vi "rsscope_core_global.vi"() -> ()   [LabVIEW 2018] (continued)
None\n\nRemote-control command(s):\nSEARch:TRIGger:HBTO:ERRor:PREamble"}, {"Level"=4, "Class Only"=FALSE, "Identifier"="RSSCOPE_ATTR_SEARCH_100BASE_T1_ERROR_CRC", "Descriptive Name"="Search 100BASE-T1 Error CRC", "Data Type"=3, "Command"="SEAR:TRIG:HBTO:ERR:CRC", "Access"=2, "Range Table"="", "Read Callback"="rsscope_FormatSearchNameBoolean_ReadCallback.vi", "Write Callback"="rsscope_FormatSearchNameBoolean_WriteCallback.vi", "Supported Models"="", "Instrument Options"="K57", "Flags"=0, "Help"="Enables / disables trigger on Cyclic Redundancy Check (CRC) error.\n\nAvailable Repeated Capabilities:\nNone\n\nRemote-control command(s):\nSEARch:TRIGger:HBTO:ERRor:CRC"}, {"Level"=4, "Class Only"=FALSE, "Identifier"="RSSCOPE_ATTR_SEARCH_100BASE_T1_ERROR_SFD", "Descriptive Name"="Search 100BASE-T1 Error SFD", "Data Type"=3, "Command"="SEAR:TRIG:HBTO:ERR:SFD", "Access"=2, "Range Table"="", "Read Callback"="rsscope_FormatSearchNameBoolean_ReadCallback.vi", "Write Callback"="rsscope_FormatSearchNameBoolean_WriteCallback.vi", "Supported Models"="", "Instrument Options"="K57", "Flags"=0, "Help"="Enables / disables search for start frame delimiter (SFD) error.\n\nAvailable Repeated Capabilities:\nNone\n\nRemote-control command(s):\nSEARch:TRIGger:HBTO:ERRor:SFD"}, {"Level"=4, "Class Only"=TRUE, "Identifier"="", "Descriptive Name"="Results", "Data Type"=0, "Command"="", "Access"=0, "Range Table"="", "Read Callback"="", "Write Callback"="", "Supported Models"="", "Instrument Options"="", "Flags"=0, "Help"="Returns the search results."}, {"Level"=5, "Class Only"=FALSE, "Identifier"="RSSCOPE_ATTR_SEARCH_100BASE_T1_FRAME_COUNT", "Descriptive Name"="Search 100BASE-T1 Frame Count", "Data Type"=0, "Command"="SEAR:RES:HBTO:FCO?", "Access"=0, "Range Table"="", "Read Callback"="rsscope_FormatSearchNameInt32_ReadCallback.vi", "Write Callback"="", "Supported Models"="", "Instrument Options"="K57", "Flags"=0, "Help"="Returns the number of decoded frames within the search result.\n\nAvailable Repeated Capabilities:\nNone\n\nRemote-control command(s):\nSEARch:RESult:HBTO:FCOunt?"}, {"Level"=3, "Class Only"=TRUE, "Identifier"="", "Descriptive Name"="1000BASE-T1", "Data Type"=0, "Command"="", "Access"=0, "Range Table"="", "Read Callback"="", "Write Callback"="", "Supported Models"="", "Instrument Options"="", "Flags"=0, "Help"="Configures 1000BASE-T1 search"}, {"Level"=4, "Class Only"=FALSE, "Identifier"="RSSCOPE_ATTR_SEARCH_1000BASE_T1_TYPE", "Descriptive Name"="Search 1000BASE-T1 Type", "Data Type"=0, "Command"="SEAR:TRIG:TBTO:TYPE", "Access"=2, "Range Table"="RsScope_rngSearch1000BASE_T1Type", "Read Callback"="rsscope_FormatSearchNameInt32_ReadCallback.vi", "Write Callback"="rsscope_FormatSearchNameInt32_WriteCallback.vi", "Supported Models"="", "Instrument Options"="K58", "Flags"=0, "Help"="Selects the type of frame to be searched for.\n\nAvailable Repeated Capabilities:\nNone\n\nRemote-control command(s):\nSEARch:TRIGger:TBTO:TYPE"}, {"Level"=4, "Class Only"=FALSE, "Identifier"="RSSCOPE_ATTR_SEARCH_1000BASE_T1_DESTINATION_ADDRESS_CONDITION", "Descriptive Name"="Search 1000BASE-T1 Destination Address Condition", "Data Type"=0, "Command"="SEAR:TRIG:TBTO:DADD:COND", "Access"=2, "Range Table"="rsscope_rngProtocolTriggerConditionStrict", "Read Callback"="rsscope_FormatSearchNameInt32_ReadCallback.vi", "Write Callback"="rsscope_FormatSearchNameInt32_WriteCallback.vi", "Supported Models"="", "Instrument Options"="K58", "Flags"=0, "Help"="Sets the condition for the destination address. You can define an exact value or a value range.\n\nAvailable Repeated Capabilities:\nNone\n\nRemote-control command(s):\nSEARch:TRIGger:TBTO:DADDress:CONDition"}, {"Level"=4, "Class Only"=FALSE, "Identifier"="RSSCOPE_ATTR_SEARCH_1000BASE_T1_DESTINATION_ADDRESS_MIN", "Descriptive Name"="Search 1000BASE-T1 Destination Address Min", "Data Type"=2, "Command"="SEAR:TRIG:TBTO:DADD:MIN", "Access"=2, "Range Table"="", "Read Callback"="rsscope_FormatSearchNameString_ReadCallback.vi", "Write Callback"="rsscope_FormatSearchNameString_WriteCallback.vi", "Supported Models"="", "Instrument Options"="K58", "Flags"=0, "Help"="Specifies the destination address bit pattern, or sets the start value of a pattern range. The string parameter accepts the bit value X (do not care).\n\nAvailable Repeated Capabilities:\nNone\n\nRemote-control command(s):\nSEARch:TRIGger:TBTO:DADDress:MIN"}, {"Level"=4, "Class Only"=FALSE, "Identifier"="RSSCOPE_ATTR_SEARCH_1000BASE_T1_DESTINATION_ADDRESS_MAX", "Descriptive Name"="Search 1000BASE-T1 Destination Address Max", "Data Type"=2, "Command"="SEAR:TRIG:TBTO:DADD:MAX", "Access"=2, "Range Table"="", "Read Callback"="rsscope_FormatSearchNameString_ReadCallback.vi", "Write Callback"="rsscope_FormatSearchNameString_WriteCallback.vi", "Supported Models"="", "Instrument Options"="K58", "Flags"=0, "Help"="Sets the end value of the destination address range if RSSCOPE_ATTR_SEARCH_1000BASE_T1_DESTINATION_ADDRESS_CONDITION is set to In Range or Out Of Range. The string parameter accepts the bit value X (do not care).\n\nAvailable Repeated Capabilities:\nNone\n\nRemote-control command(s):\nSEARch:TRIGger:TBTO:DADDress:MAX"}, {"Level"=4, "Class Only"=FALSE, "Identifier"="RSSCOPE_ATTR_SEARCH_1000BASE_T1_SOURCE_ADDRESS_CONDITION", "Descriptive Name"="Search 1000BASE-T1 Source Address Condition", "Data Type"=0, "Command"="SEAR:TRIG:TBTO:SADD:COND", "Access"=2, "Range Table"="rsscope_rngProtocolTriggerConditionStrict", "Read Callback"="rsscope_FormatSearchNameInt32_ReadCallback.vi", "Write Callback"="rsscope_FormatSearchNameInt32_WriteCallback.vi", "Supported Models"="", "Instrument Options"="K58", "Flags"=0, "Help"="Sets the condition for the source address. You can define an exact value or a value range.\n\nAvailable Repeated Capabilities:\nNone\n\nRemote-control command(s):\nSEARch:TRIGger:TBTO:SADDress:CONDition"}, {"Level"=4, "Class Only"=FALSE, "Identifier"="RSSCOPE_ATTR_SEARCH_1000BASE_T1_SOURCE_ADDRESS_MIN", "Descriptive Name"="Search 1000BASE-T1 Source Address Min", "Data Type"=2, "Command"="SEAR:TRIG:TBTO:SADD:MIN", "Access"=2, "Range Table"="", "Read Callback"="rsscope_FormatSearchNameString_ReadCallback.vi", "Write Callback"="rsscope_FormatSearchNameString_WriteCallback.vi", "Supported Models"="", "Instrument Options"="K58", "Flags"=0, "Help"="Specifies the source address bit pattern, or sets the start value of a pattern range. The string parameter accepts the bit value X (do not care).\n\nAvailable Repeated Capabilities:\nNone\n\nRemote-control command(s):\nSEARch:TRIGger:TBTO:SADDress:MIN"}, {"Level"=4, "Class Only"=FALSE, "Identifier"="RSSCOPE_ATTR_SEARCH_1000BASE_T1_SOURCE_ADDRESS_MAX", "Descriptive Name"="Search 1000BASE-T1 Source Address Max", "Data Type"=2, "Command"="SEAR:TRIG:TBTO:SADD:MAX", "Access"=2, "Range Table"="", "Read Callback"="rsscope_FormatSearchNameString_ReadCallback.vi", "Write Callback"="rsscope_FormatSearchNameString_WriteCallback.vi", "Supported Models"="", "Instrument Options"="K58", "Flags"=0, "Help"="Sets the end value of the source address range if RSSCOPE_ATTR_SEARCH_1000BASE_T1_SOURCE_ADDRESS_CONDITION is set to In Range or Out Of Range. The string parameter accepts the bit value X (do not care).\n\nAvailable Repeated Capabilities:\nNone\n\nRemote-control command(s):\nSEARch:TRIGger:TBTO:SADDress:MAX"}, {"Level"=4, "Class Only"=FALSE, "Identifier"="RSSCOPE_ATTR_SEARCH_1000BASE_T1_LENGTH_TYPE_CONDITION", "Descriptive Name"="Search 1000BASE-T1 Length Type Condition", "Data Type"=0, "Command"="SEAR:TRIG:TBTO:LENG:COND", "Access"=2, "Range Table"="rsscope_rngProtocolTriggerConditionStrict", "Read Callback"="rsscope_FormatSearchNameInt32_ReadCallback.vi", "Write Callback"="rsscope_FormatSearchNameInt32_WriteCallback.vi", "Supported Models"="", "Instrument Options"="K58", "Flags"=0, "Help"="Sets the condition for the length/type. You can define an exact value or a value range.\n\nAvailable Repeated Capabilities:\nNone\n\nRemote-control command(s):\nSEARch:TRIGger:TBTO:LENGth:CONDition"}, {"Level"=4, "Class Only"=FALSE, "Identifier"="RSSCOPE_ATTR_SEARCH_1000BASE_T1_LENGTH_TYPE_MIN", "Descriptive Name"="Search 1000BASE-T1 Length Type Min", "Data Type"=2, "Command"="SEAR:TRIG:TBTO:LENG:MIN", "Access"=2, "Range Table"="", "Read Callback"="rsscope_FormatSearchNameString_ReadCallback.vi", "Write Callback"="rsscope_FormatSearchNameString_WriteCallback.vi", "Supported Models"="", "Instrument Options"="K58", "Flags"=0, "Help"="Specifies the length/ type bit pattern, or sets the start value of a pattern range. The string parameter accepts the bit value X (do not care).\n\nAvailable Repeated Capabilities:\nNone\n\nRemote-control command(s):\nSEARch:TRIGger:TBTO:LENGth:MIN"}, {"Level"=4, "Class Only"=FALSE, "Identifier"="RSSCOPE_ATTR_SEARCH_1000BASE_T1_LENGTH_TYPE_MAX", "Descriptive Name"="Search 1000BASE-T1 Length Type Max", "Data Type"=2, "Command"="SEAR:TRIG:TBTO:LENG:MAX", "Access"=2, "Range Table"="", "Read Callback"="rsscope_FormatSearchNameString_ReadCallback.vi", "Write Callback"="rsscope_FormatSearchNameString_WriteCallback.vi", "Supported Models"="", "Instrument Options"="K58", "Flags"=0, "Help"="Sets the end value of the length/type range if RSSCOPE_ATTR_SEARCH_1000BASE_T1_TYPE_LENGTH_CONDITION is set to In Range or Out Of Range. The string parameter accepts the bit value X (do not care).\n\nAvailable Repeated Capabilities:\nNone\n\nRemote-control command(s):\nSEARch:TRIGger:TBTO:LENGth:MAX"}, {"Level"=4, "Class Only"=FALSE, "Identifier"="RSSCOPE_ATTR_SEARCH_1000BASE_T1_FRAME_CHECK_CRC_CONDITION", "Descriptive Name"="Search 1000BASE-T1 Frame Check CRC Condition", "Data Type"=0, "Command"="SEAR:TRIG:TBTO:CRC:COND", "Access"=2, "Range Table"="rsscope_rngProtocolTriggerConditionStrict", "Read Callback"="rsscope_FormatSearchNameInt32_ReadCallback.vi", "Write Callback"="rsscope_FormatSearchNameInt32_WriteCallback.vi", "Supported Models"="", "Instrument Options"="K58", "Flags"=0, "Help"="Sets the condition for the frame check. You can define an exact value or a value range.\n\nAvailable Repeated Capabilities:\nNone\n\nRemote-control command(s):\nSEARch:TRIGger:TBTO:CRC:CONDition"}, {"Level"=4, "Class Only"=FALSE, "Identifier"="RSSCOPE_ATTR_SEARCH_1000BASE_T1_FRAME_CHECK_CRC_MIN", "Descriptive Name"="Search 1000BASE-T1 Frame Check CRC Min", "Data Type"=2, "Command"="SEAR:TRIG:TBTO:CRC:MIN", "Access"=2, "Range Table"="", "Read Callback"="rsscope_FormatSearchNameString_ReadCallback.vi", "Write Callback"="rsscope_FormatSearchNameString_WriteCallback.vi", "Supported Models"="", "Instrument Options"="K58", "Flags"=0, "Help"="Specifies the frame check bit pattern, or sets the start value of a pattern range. The string parameter accepts the bit value X (do not care).\n\nAvailable Repeated Capabilities:\nNone\n\nRemote-control command(s):\nSEARch:TRIGger:TBTO:CRC:MIN"}, {"Level"=4, "Class Only"=FALSE, "Identifier"="RSSCOPE_ATTR_SEARCH_1000BASE_T1_FRAME_CHECK_CRC_MAX", "Descriptive Name"="Search 1000BASE-T1 Frame Check CRC Max", "Data Type"=2, "Command"="SEAR:TRIG:TBTO:CRC:MAX", "Access"=2, "Range Table"="", "Read Callback"="rsscope_FormatSearchNameString_ReadCallback.vi", "Write Callback"="rsscope_FormatSearchNameString_WriteCallback.vi", "Supported Models"="", "Instrument Options"="K58", "Flags"=0, "Help"="Sets the end value of the frame check range if RSSCOPE_ATTR_SEARCH_1000BASE_T1_CRC_CONDITION is set to In Range or Out Of Range. The string parameter accepts the bit value X (do not care).\n\nAvailable Repeated Capabilities:\nNone\n\nRemote-control command(s):\nSEARch:TRIGger:TBTO:CRC:MAX"}, {"Level"=4, "Class Only"=FALSE, "Identifier"="RSSCOPE_ATTR_SEARCH_1000BASE_T1_DATA_CONDITION", "Descriptive Name"="Search 1000BASE-T1 Data Condition", "Data Type"=0, "Command"="SEAR:TRIG:TBTO:DATA:DCON", "Access"=2, "Range Table"="rsscope_rngProtocolTriggerConditionStrict", "Read Callback"="rsscope_FormatSearchNameInt32_ReadCallback.vi", "Write Callback"="rsscope_FormatSearchNameInt32_WriteCallback.vi", "Supported Models"="", "Instrument Options"="K58", "Flags"=0, "Help"="Sets the condition for the data. You can define an exact value or a value range.\n\nAvailable Repeated Capabilities:\nNone\n\nRemote-control command(s):\nSEARch:TRIGger:TBTO:DATA:DCONdition"}, {"Level"=4, "Class Only"=FALSE, "Identifier"="RSSCOPE_ATTR_SEARCH_1000BASE_T1_DATA_MIN", "Descriptive Name"="Search 1000BASE-T1 Data Min", "Data Type"=2, "Command"="SEAR:TRIG:TBTO:DATA:DMIN", "Access"=2, "Range Table"="", "Read Callback"="rsscope_FormatSearchNameString_ReadCallback.vi", "Write Callback"="rsscope_FormatSearchNameString_WriteCallback.vi", "Supported Models"="", "Instrument Options"="K58", "Flags"=0, "Help"="Specifies the data bit pattern, or sets the start value of a pattern range. The string parameter accepts the bit value X (do not care).\n\nAvailable Repeated Capabilities:\nNone\n\nRemote-control command(s):\nSEARch:TRIGger:TBTO:DATA:DMIN"}, {"Level"=4, "Class Only"=FALSE, "Identifier"="RSSCOPE_ATTR_SEARCH_1000BASE_T1_DATA_MAX", "Descriptive Name"="Search 1000BASE-T1 Data Max", "Data Type"=2, "Command"="SEAR:TRIG:TBTO:DATA:DMAX", "Access"=2, "Range Table"="", "Read Callback"="rsscope_FormatSearchNameString_ReadCallback.vi", "Write Callback"="rsscope_FormatSearchNameString_WriteCallback.vi", "Supported Models"="", "Instrument Options"="K58", "Flags"=0, "Help"="Sets the end value of the data range if RSSCOPE_ATTR_SEARCH_1000BASE_T1_DATA_CONDITION is set to In Range or Out Of Range. The string parameter accepts the bit value X (do not care).\n\nAvailable Repeated Capabilities:\nNone\n\nRemote-control command(s):\nSEARch:TRIGger:TBTO:DATA:DMAX"}, {"Level"=4, "Class Only"=FALSE, "Identifier"="RSSCOPE_ATTR_SEARCH_1000BASE_T1_INDEX_CONDITION", "Descriptive Name"="Search 1000BASE-T1 Index Condition", "Data Type"=0, "Command"="SEAR:TRIG:TBTO:DATA:ICON", "Access"=2, "Range Table"="rsscope_rngProtocolTriggerConditionStrict", "Read Callback"="rsscope_FormatSearchNameInt32_ReadCallback.vi", "Write Callback"="rsscope_FormatSearchNameInt32_WriteCallback.vi", "Supported Models"="", "Instrument Options"="K58", "Flags"=0, "Help"="Sets the search condition for the index. You can define an exact value or a value range.\n\nAvailable Repeated Capabilities:\nNone\n\nRemote-control command(s):\nSEARch:TRIGger:TBTO:DATA:ICONdition"}, {"Level"=4, "Class Only"=FALSE, "Identifier"="RSSCOPE_ATTR_SEARCH_1000BASE_T1_INDEX_MIN", "Descriptive Name"="Search 1000BASE-T1 Index Min", "Data Type"=0, "Command"="SEAR:TRIG:TBTO:DATA:IMIN", "Access"=2, "Range Table"="RsScope_rng1000BASET1Index", "Read Callback"="rsscope_FormatSearchNameInt32_ReadCallback.vi", "Write Callback"="rsscope_FormatSearchNameInt32_WriteCallback.vi", "Supported Models"="", "Instrument Options"="K58", "Flags"=0, "Help"="Specifies the index bit pattern, or sets the start value of a pattern range.\n\nAvailable Repeated Capabilities:\nNone\n\nRemote-control command(s):\nSEARch:TRIGger:TBTO:DATA:IMIN"}, {"Level"=4, "Class Only"=FALSE, "Identifier"="RSSCOPE_ATTR_SEARCH_1000BASE_T1_INDEX_MAX", "Descriptive Name"="Search 1000BASE-T1 Index Max", "Data Type"=0, "Command"="SEAR:TRIG:TBTO:DATA:IMAX", "Access"=2, "Range Table"="RsScope_rng1000BASET1Index", "Read Callback"="rsscope_FormatSearchNameInt32_ReadCallback.vi", "Write Callback"="rsscope_FormatSearchNameInt32_WriteCallback.vi", "Supported Models"="", "Instrument Options"="K58", "Flags"=0, "Help"="Sets the end value of the index range to be searched for, if RSSCOPE_ATTR_SEARCH_1000BASE_T1_INDEX_CONDITION is set to In Range or Out Of Range.\n\nAvailable Repeated Capabilities:\nNone\n\nRemote-control command(s):\nSEARch:TRIGger:TBTO:DATA:IMAX"}, {"Level"=4, "Class Only"=FALSE, "Identifier"="RSSCOPE_ATTR_SEARCH_1000BASE_T1_ERROR_RS_FEC", "Descriptive Name"="Search 1000BASE-T1 Error RS-FEC", "Data Type"=3, "Command"="SEAR:TRIG:TBTO:ERR:FEC", "Access"=2, "Range Table"="", "Read Callback"="rsscope_FormatSearchNameBoolean_ReadCallback.vi", "Write Callback"="rsscope_FormatSearchNameBoolean_WriteCallback.vi", "Supported Models"="", "Instrument Options"="K58", "Flags"=0, "Help"="Enables search for RS-FEC errors.\n\nAvailable Repeated Capabilities:\nNone\n\nRemote-control command(s):\nSEARch:TRIGger:TBTO:ERRor:FEC"}, {"Level"=4, "Class Only"=FALSE, "Identifier"="RSSCOPE_ATTR_SEARCH_1000BASE_T1_ERROR_CRC", "Descriptive Name"="Search 1000BASE-T1 Error CRC", "Data Type"=3, "Command"="SEAR:TRIG:TBTO:ERR:CRC", "Access"=2, "Range Table"="", "Read Callback"="rsscope_FormatSearchNameBoolean_ReadCallback.vi", "Write Callback"="rsscope_FormatSearchNameBoolean_WriteCallback.vi", "Supported Models"="", "Instrument Options"="K58", "Flags"=0, "Help"="Enables search for cyclic redundancy check (CRC) error.\n\nAvailable Repeated Capabilities:\nNone\n\nRemote-control command(s):\nSEARch:TRIGger:TBTO:ERRor:CRC"}, {"Level"=4, "Class Only"=FALSE, "Identifier"="RSSCOPE_ATTR_SEARCH_1000BASE_T1_ERROR_OUT_OF_RANGE", "Descriptive Name"="Search 1000BASE-T1 Error Out Of Range", "Data Type"=3, "Command"="SEAR:TRIG:TBTO:ERR:OOR", "Access"=2, "Range Table"="", "Read Callback"="rsscope_FormatSearchNameBoolean_ReadCallback.vi", "Write Callback"="rsscope_FormatSearchNameBoolean_WriteCallback.vi", "Supported Models"="", "Instrument Options"="K58", "Flags"=0, "Help"="Enables search for values that are out of range.\n\nAvailable Repeated Capabilities:\nNone\n\nRemote-control command(s):\nSEARch:TRIGger:TBTO:ERRor:OOR"}, {"Level"=4, "Class Only"=FALSE, "Identifier"="RSSCOPE_ATTR_SEARCH_1000BASE_T1_ERROR_ZERO_TERNARY_SYMBOL", "Descriptive Name"="Search 1000BASE-T1 Error Zero Ternary Symbol", "Data Type"=3, "Command"="SEAR:TRIG:TBTO:ERR:ZERO", "Access"=2, "Range Table"="", "Read Callback"="rsscope_FormatSearchNameBoolean_ReadCallback.vi", "Write Callback"="rsscope_FormatSearchNameBoolean_WriteCallback.vi", "Supported Models"="", "Instrument Options"="K58", "Flags"=0, "Help"="Enables search for zero ternary symbol pairs error.\n\nAvailable Repeated Capabilities:\nNone\n\nRemote-control command(s):\nSEARch:TRIGger:TBTO:ERRor:ZERO"}, {"Level"=4, "Class Only"=TRUE, "Identifier"="", "Descriptive Name"="Results", "Data Type"=0, "Command"="", "Access"=0, "Range Table"="", "Read Callback"="", "Write Callback"="", "Supported Models"="", "Instrument Options"="", "Flags"=0, "Help"="Returns the search results."}, {"Level"=5, "Class Only"=FALSE, "Identifier"="RSSCOPE_ATTR_SEARCH_1000BASE_T1_FRAME_COUNT", "Descriptive Name"="Search 1000BASE-T1 Frame Count", "Data Type"=0, "Command"="SEAR:RES:TBTO:FCO?", "Access"=0, "Range Table"="", "Read Callback"="rsscope_FormatSearchNameInt32_ReadCallback.vi", "Write Callback"="", "Supported Models"="", "Instrument Options"="K58", "Flags"=0, "Help"="Returns the number of decoded frames within the search result.\n\nAvailable Repeated Capabilities:\nNone\n\nRemote-control command(s):\nSEARch:RESult:TBTO:FCOunt?"}, {"Level"=5, "Class Only"=FALSE, "Identifier"="RSSCOPE_ATTR_SEARCH_1000BASE_T1_SELECTED_FRAME", "Descriptive Name"="Search 1000BASE-T1 Selected Frame", "Data Type"=0, "Command"="", "Access"=2, "Range Table"="", "Read Callback"="", "Write Callback"="", "Supported Models"="", "Instrument Options"="K58", "Flags"=0, "Help"="Sets the selector for the Frame repeated capability.\n\nAvailable Repeated Capabilities:\nNone\n\nRemote-control command(s):\n"}, {"Level"=5, "Class Only"=FALSE, "Identifier"="RSSCOPE_ATTR_SEARCH_1000BASE_T1_FRAME_STATUS", "Descriptive Name"="Search 1000BASE-T1 Frame Status", "Data Type"=0, "Command"="SEAR:RES:TBTO:FRAM<Frame>:STAT?", "Access"=0, "Range Table"="RsScope_rngProtocol1000BASE_T1FrameStatus", "Read Callback"="rsscope_FormatSearchNameTBTOFrameInt32_ReadCallback.vi", "Write Callback"="", "Supported Models"="", "Instrument Options"="K58", "Flags"=0, "Help"="Returns the state of the frame within the search result.\n\nAvailable Repeated Capabilities:\nNone\n\nRemote-control command(s):\nSEARch:RESult:TBTO:FRAMe<m>:STATe?"}, {"Level"=5, "Class Only"=FALSE, "Identifier"="RSSCOPE_ATTR_SEARCH_1000BASE_T1_FRAME_START_TIME", "Descriptive Name"="Search 1000BASE-T1 Frame Start Time", "Data Type"=1, "Command"="SEAR:RES:TBTO:FRAM<Frame>:STAR?", "Access"=0, "Range Table"="", "Read Callback"="rsscope_FormatSearchNameTBTOFrameReal64_ReadCallback.vi", "Write Callback"="", "Supported Models"="", "Instrument Options"="K58", "Flags"=0, "Help"="Returns the start time of the selected frame within the search result.\n\nAvailable Repeated Capabilities:\nNone\n\nRemote-control command(s):\nSEARch:RESult:TBTO:FRAMe<m>:STARt?"}, {"Level"=5, "Class Only"=FALSE, "Identifier"="RSSCOPE_ATTR_SEARCH_1000BASE_T1_FRAME_STOP_TIME", "Descriptive Name"="Search 1000BASE-T1 Frame Stop Time", "Data Type"=1, "Command"="SEAR:RES:TBTO:FRAM<Frame>:STOP?", "Access"=0, "Range Table"="", "Read Callback"="rsscope_FormatSearchNameTBTOFrameReal64_ReadCallback.vi", "Write Callback"="", "Supported Models"="", "Instrument Options"="K58", "Flags"=0, "Help"="Returns the end time of the selected frame within the search result.\n\nAvailable Repeated Capabilities:\nNone\n\nRemote-control command(s):\nSEARch:RESult:TBTO:FRAMe<m>:STOP?"}, {"Level"=5, "Class Only"=FALSE, "Identifier"="RSSCOPE_ATTR_SEARCH_1000BASE_T1_FRAME_DESTINATION", "Descriptive Name"="Search 1000BASE-T1 Frame Destination", "Data Type"=2, "Command"="SEAR:RES:TBTO:FRAM<Frame>:DEST?", "Access"=0, "Range Table"="", "Read Callback"="rsscope_FormatSearchNameTBTOFrameString_ReadCallback.vi", "Write Callback"="", "Supported Models"="", "Instrument Options"="K58", "Flags"=0, "Help"="Returns the destination address of the selected frame within the search result.\n\nAvailable Repeated Capabilities:\nNone\n\nRemote-control command(s):\nSEARch:RESult:TBTO:FRAMe<m>:DESTaddress?"}, {"Level"=5, "Class Only"=FALSE, "Identifier"="RSSCOPE_ATTR_SEARCH_1000BASE_T1_FRAME_DESTINATION_SYMBOLS", "Descriptive Name"="Search 1000BASE-T1 Frame Destination Symbols", "Data Type"=2, "Command"="SEAR:RES:TBTO:FRAM<Frame>:DSYM?", "Access"=0, "Range Table"="", "Read Callback"="rsscope_FormatSearchNameTBTOFrameString_ReadCallback.vi", "Write Callback"="", "Supported Models"="", "Instrument Options"="K58", "Flags"=0, "Help"="Returns the destination symbols of the selected frame within the search result.\n\nAvailable Repeated Capabilities:\nNone\n\nRemote-control command(s):\nSEARch:RESult:TBTO:FRAMe<m>:DSYMbol?"}, {"Level"=5, "Class Only"=FALSE, "Identifier"="RSSCOPE_ATTR_SEARCH_1000BASE_T1_FRAME_SOURCE", "Descriptive Name"="Search 1000BASE-T1 Frame Source", "Data Type"=2, "Command"="SEAR:RES:TBTO:FRAM<Frame>:SRC?", "Access"=0, "Range Table"="", "Read Callback"="rsscope_FormatSearchNameTBTOFrameString_ReadCallback.vi", "Write Callback"="", "Supported Models"="", "Instrument Options"="K58", "Flags"=0, "Help"="Returns the source address of the selected frame within the search result.\n\nAvailable Repeated Capabilities:\nNone\n\nRemote-control command(s):\nSEARch:RESult:TBTO:FRAMe<m>:SRCaddress?"}, {"Level"=5, "Class Only"=FALSE, "Identifier"="RSSCOPE_ATTR_SEARCH_1000BASE_T1_FRAME_SOURCE_SYMBOLS", "Descriptive Name"="Search 1000BASE-T1 Frame Source Symbols", "Data Type"=2, "Command"="SEAR:RES:TBTO:FRAM<Frame>:SSYM?", "Access"=0, "Range Table"="", "Read Callback"="rsscope_FormatSearchNameTBTOFrameString_ReadCallback.vi", "Write Callback"="", "Supported Models"="", "Instrument Options"="K58", "Flags"=0, "Help"="Returns the source symbols of the selected frame within the search result.\n\nAvailable Repeated Capabilities:\nNone\n\nRemote-control command(s):\nSEARch:RESult:TBTO:FRAMe<m>:SSYMbol?"}, {"Level"=5, "Class Only"=FALSE, "Identifier"="RSSCOPE_ATTR_SEARCH_1000BASE_T1_FRAME_DATA_STRING", "Descriptive Name"="Search 1000BASE-T1 Frame Data String", "Data Type"=2, "Command"="SEAR:RES:TBTO:FRAM<Frame>:DATA?", "Access"=0, "Range Table"="", "Read Callback"="rsscope_FormatSearchNameTBTOFrameString_ReadCallback.vi", "Write Callback"="", "Supported Models"="", "Instrument Options"="K58", "Flags"=0, "Help"="Returns the data for the selected frame.\n\nAvailable Repeated Capabilities:\nNone\n\nRemote-control command(s):\nSEARch:RESult:TBTO:FRAMe<m>:DATA?"}, {"Level"=5, "Class Only"=FALSE, "Identifier"="RSSCOPE_ATTR_SEARCH_1000BASE_T1_FRAME_CRC", "Descriptive Name"="Search 1000BASE-T1 Frame CRC", "Data Type"=5, "Command"="SEAR:RES:TBTO:FRAM<Frame>:CRC?", "Access"=0, "Range Table"="", "Read Callback"="rsscope_FormatSearchNameTBTOFrameInt64_ReadCallback.vi", "Write Callback"="", "Supported Models"="", "Instrument Options"="K58", "Flags"=0, "Help"="Returns the CRC checksum of the selected frame within the search result.\n\nAvailable Repeated Capabilities:\nNone\n\nRemote-control command(s):\nSEARch:RESult:TBTO:FRAMe<m>:CRC?"}, {"Level"=5, "Class Only"=FALSE, "Identifier"="RSSCOPE_ATTR_SEARCH_1000BASE_T1_FRAME_LENGTH_TYPE", "Descriptive Name"="Search 1000BASE-T1 Frame Length Type", "Data Type"=0, "Command"="SEAR:RES:TBTO:FRAM<Frame>:TYPE?", "Access"=0, "Range Table"="", "Read Callback"="rsscope_FormatSearchNameTBTOFrameInt32_ReadCallback.vi", "Write Callback"="", "Supported Models"="", "Instrument Options"="K58", "Flags"=0, "Help"="Returns the value of length / type field of the selected frame within the search result.\n\nAvailable Repeated Capabilities:\nNone\n\nRemote-control command(s):\nSEARch:RESult:TBTO:FRAMe<m>:TYPE?"}, {"Level"=5, "Class Only"=FALSE, "Identifier"="RSSCOPE_ATTR_SEARCH_1000BASE_T1_FRAME_TYPE", "Descriptive Name"="Search 1000BASE-T1 Frame Type", "Data Type"=0, "Command"="SEAR:RES:TBTO:FRAM<Frame>:FTYP?", "Access"=0, "Range Table"="RsScope_rngProtocol1000BASE_T1FrameType", "Read Callback"="rsscope_FormatSearchNameTBTOFrameInt32_ReadCallback.vi", "Write Callback"="", "Supported Models"="", "Instrument Options"="K58", "Flags"=0, "Help"="Returns the type of frame for the selected frame within the search result.\n\nAvailable Repeated Capabilities:\nNone\n\nRemote-control command(s):\nSEARch:RESult:TBTO:FRAMe<m>:FTYPe?"}, {"Level"=5, "Class Only"=FALSE, "Identifier"="RSSCOPE_ATTR_SEARCH_1000BASE_T1_FRAME_NUMBER_OF_WORDS", "Descriptive Name"="Search 1000BASE-T1 Frame Number Of Words", "Data Type"=5, "Command"="SEAR:RES:TBTO:FRAM<Frame>:NUMW?", "Access"=0, "Range Table"="", "Read Callback"="rsscope_FormatSearchNameTBTOFrameInt64_ReadCallback.vi", "Write Callback"="", "Supported Models"="", "Instrument Options"="K58", "Flags"=0, "Help"="Returns the number of decoded words for the selected frame within the search result.\n\nAvailable Repeated Capabilities:\nNone\n\nRemote-control command(s):\nSEARch:RESult:TBTO:FRAMe<m>:NUMWords?"}, {"Level"=5, "Class Only"=FALSE, "Identifier"="RSSCOPE_ATTR_SEARCH_1000BASE_T1_SELECTED_WORD", "Descriptive Name"="Search 1000BASE-T1 Selected Word", "Data Type"=5, "Command"="", "Access"=2, "Range Table"="", "Read Callback"="", "Write Callback"="", "Supported Models"="", "Instrument Options"="K58", "Flags"=0, "Help"="Sets the selector for the Word  repeated capability.\n\nAvailable Repeated Capabilities:\nNone\n\nRemote-control command(s):\n"}, {"Level"=5, "Class Only"=FALSE, "Identifier"="RSSCOPE_ATTR_SEARCH_1000BASE_T1_FRAME_WORD_TYPE", "Descriptive Name"="Search 1000BASE-T1 Frame Word Type", "Data Type"=2, "Command"="SEAR:RES:TBTO:FRAM<Frame>:WORD<Word>:TYPE?", "Access"=0, "Range Table"="", "Read Callback"="rsscope_FormatSearchNameTBTOWordString_ReadCallback.vi", "Write Callback"="", "Supported Models"="", "Instrument Options"="K58", "Flags"=0, "Help"="Returns the data type of the selected word within the search result.\n\nAvailable Repeated Capabilities:\nNone\n\nRemote-control command(s):\nSEARch:RESult:TBTO:FRAMe<m>:WORD<n>:TYPE?"}, {"Level"=5, "Class Only"=FALSE, "Identifier"="RSSCOPE_ATTR_SEARCH_1000BASE_T1_FRAME_WORD_VALUE", "Descriptive Name"="Search 1000BASE-T1 Frame Word Value", "Data Type"=0, "Command"="SEAR:RES:TBTO:FRAM<Frame>:WORD<Word>:VAL?", "Access"=0, "Range Table"="", "Read Callback"="rsscope_FormatSearchNameTBTOWordInt32_ReadCallback.vi", "Write Callback"="", "Supported Models"="", "Instrument Options"="K58", "Flags"=0, "Help"="Returns the data value of the selected word within the search result.\n\nAvailable Repeated Capabilities:\nNone\n\nRemote-control command(s):\nSEARch:RESult:TBTO:FRAMe<m>:WORD<n>:VALue?"}, {"Level"=5, "Class Only"=FALSE, "Identifier"="RSSCOPE_ATTR_SEARCH_1000BASE_T1_FRAME_WORD_VALUE_STRING", "Descriptive Name"="Search 1000BASE-T1 Frame Word Value String", "Data Type"=2, "Command"="SEAR:RES:TBTO:FRAM<Frame>:WORD<Word>:VSTR?", "Access"=0, "Range Table"="", "Read Callback"="rsscope_FormatSearchNameTBTOWordString_ReadCallback.vi", "Write Callback"="", "Supported Models"="", "Instrument Options"="K58", "Flags"=0, "Help"="Returns the string equivalent of data value for the selected cell.\n\nAvailable Repeated Capabilities:\nNone\n\nRemote-control command(s):\nSEARch:RESult:TBTO:FRAMe<m>:WORD<n>:VSTR?"}, {"Level"=1, "Class Only"=TRUE, "Identifier"="", "Descriptive Name"="Protocols", "Data Type"=0, "Command"="", "Access"=0, "Range Table"="", "Read Callback"="", "Write Callback"="", "Supported Models"="", "Instrument Options"="", "Flags"=0, "Help"="Analyze the following serial protocols:\n\n- SPI (Serial Peripheral Interface) - decoding requires option R&S RTO-K1\n- I2C (Inter-Integrated circuit bus) - decoding requires option R&S RTO-K1\n- UART/RS232 (EIA-232 serial interface) - decoding requires option R&S RTO-K2\n\nTriggering on SPI, I2C and UART is available with the main R&S RTO without any options."}, {"Level"=2, "Class Only"=FALSE, "Identifier"="RSSCOPE_ATTR_PROTOCOL_STATE", "Descriptive Name"="Protocol State", "Data Type"=3, "Command"="BUS{SerialBus}:STAT", "Access"=2, "Range Table"="", "Read Callback"="", "Write Callback"="", "Supported Models"="", "Instrument Options"="", "Flags"=0, "Help"="Switches the protocol display on or off.\n\nAvailable Repeated Capabilities:\nSerialBus: SB1, SB2, SB3, SB4\r\n\nRemote-control command(s):\nBUS<m>[:STATe]"}, {"Level"=2, "Class Only"=FALSE, "Identifier"="RSSCOPE_ATTR_PROTOCOL_TYPE", "Descriptive Name"="Protocol Type", "Data Type"=0, "Command"="BUS{SerialBus}:TYPE", "Access"=2, "Range Table"="rsscope_rngProtocolType", "Read Callback"="", "Write Callback"="", "Supported Models"="", "Instrument Options"="", "Flags"=0, "Help"="Defines the bus or protocol type for analysis.\n\nNote(s):\n\n1) MIL1553 and ARINC429 are not supported on RTE\n\nAvailable Repeated Capabilities:\nSerialBus: SB1, SB2, SB3, SB4\r\n\nRemote-control command(s):\nBUS<m>:TYPE"}, {"Level"=2, "Class Only"=FALSE, "Identifier"="RSSCOPE_ATTR_PROTOCOL_LABEL", "Descriptive Name"="Protocol Label", "Data Type"=2, "Command"="BUS{SerialBus}:LAB", "Access"=2, "Range Table"="", "Read Callback"="", "Write Callback"="", "Supported Models"="", "Instrument Options"="", "Flags"=0, "Help"="Defines a label to be displayed with the bus.\n\nAvailable Repeated Capabilities:\nSerialBus: SB1, SB2, SB3, SB4\r\n\nRemote-control command(s):\nBUS<m>:LABel"}, {"Level"=2, "Class Only"=FALSE, "Identifier"="RSSCOPE_ATTR_PROTOCOL_DISPLAY_RESULT_TABLE", "Descriptive Name"="Protocol Display Result Table", "Data Type"=3, "Command"="BUS{SerialBus}:RES", "Access"=2, "Range Table"="", "Read Callback"="", "Write Callback"="", "Supported Models"="", "Instrument Options"="", "Flags"=0, "Help"="Opens a table with decoded data of the serial signal. The function requires the option for the analyzed protocol.\n\nAvailable Repeated Capabilities:\nSerialBus: SB1, SB2, SB3, SB4\r\n\nRemote-control command(s):\nBUS<m>:RESult"}, {"Level"=2, "Class Only"=FALSE, "Identifier"="RSSCOPE_ATTR_PROTOCOL_RESULT_TABLE_ZOOM_COUPLING_ENABLED", "Descriptive Name"="Protocol Result Table Zoom Coupling Enabled", "Data Type"=3, "Command"="BUS{SerialBus}:ZCO", "Access"=2, "Range Table"="", "Read Callback"="", "Write Callback"="", "Supported Models"="", "Instrument Options"="", "Flags"=0, "Help"="If enabled, the protocol decode zoom and result table are synchronized.\n\nAvailable Repeated Capabilities:\nSerialBus: SB1, SB2, SB3, SB4\r\n\nRemote-control command(s):\nBUS<m>:ZCOupling"}, {"Level"=2, "Class Only"=FALSE, "Identifier"="RSSCOPE_ATTR_PROTOCOL_RESULT_TABLE_POSITION", "Descriptive Name"="Protocol Result Table Position", "Data Type"=0, "Command"="DISP:RES:DEP", "Access"=2, "Range Table"="RsScope_rngDisplayResultTableDefaultPosition", "Read Callback"="", "Write Callback"="", "Supported Models"="", "Instrument Options"="", "Flags"=0, "Help"="Defines the position of the protocol decode result table on the screen.\n\nAvailable Repeated Capabilities:\nNone\n\nRemote-control command(s):\nDISPlay:RESultboxes:DEPosition"}, {"Level"=2, "Class Only"=FALSE, "Identifier"="RSSCOPE_ATTR_PROTOCOL_SHOW_THRESHOLD_LINES", "Descriptive Name"="Protocol Show Threshold Lines", "Data Type"=3, "Command"="BUS{SerialBus}:THR", "Access"=2, "Range Table"="", "Read Callback"="", "Write Callback"="", "Supported Models"="", "Instrument Options"="", "Flags"=0, "Help"="If ON, the threshold levels are displayed in the diagram.\n\nAvailable Repeated Capabilities:\nSerialBus: SB1, SB2, SB3, SB4\r\n\nRemote-control command(s):\nBUS<m>:THReshold"}, {"Level"=2, "Class Only"=FALSE, "Identifier"="RSSCOPE_ATTR_PROTOCOL_DATA_FORMAT", "Descriptive Name"="Protocol Data Format", "Data Type"=0, "Command"="BUSF", "Access"=2, "Range Table"="rsscope_rngProtocolDataFormat", "Read Callback"="", "Write Callback"="", "Supported Models"="", "Instrument Options"="", "Flags"=0, "Help"="Sets the data format for decoded data values in the 'Decode results' box and on the display of the decoded signal.\n\nAvailable Repeated Capabilities:\nNone\n\nRemote-control command(s):\nBUSFormat"}, {"Level"=2, "Class Only"=FALSE, "Identifier"="RSSCOPE_ATTR_PROTOCOL_SHOW_DETAILS", "Descriptive Name"="Protocol Show Details", "Data Type"=3, "Command"="BUS{SerialBus}:RESD", "Access"=2, "Range Table"="", "Read Callback"="", "Write Callback"="", "Supported Models"="", "Instrument Options"="", "Flags"=0, "Help"="Shows detailed information for the frames. The attribute is relevant for FlexRay, D-PHY, M-PHY, Ethernet, CXPI, and Custom\nprotocols.\n\nAvailable Repeated Capabilities:\nSerialBus: SB1, SB2, SB3, SB4\r\n\nRemote-control command(s):\nBUS<m>:RESDetail"}, {"Level"=2, "Class Only"=FALSE, "Identifier"="RSSCOPE_ATTR_PROTOCOL_BUS_DATA_FORMAT", "Descriptive Name"="Protocol Bus Data Format", "Data Type"=0, "Command"="BUS{SerialBus}:FORM", "Access"=2, "Range Table"="rsscope_rngProtocolDataFormat", "Read Callback"="", "Write Callback"="", "Supported Models"="", "Instrument Options"="", "Flags"=0, "Help"="Sets the number format for decoded data values of the indicated bus. It defines the format in the 'Decode table' and in the combs of the decoded signal.\n\nAvailable Repeated Capabilities:\nSerialBus: SB1, SB2, SB3, SB4\r\n\nRemote-control command(s):\nBUS<m>:FORMat"}, {"Level"=2, "Class Only"=FALSE, "Identifier"="RSSCOPE_ATTR_PROTOCOL_LABEL_LIST", "Descriptive Name"="Protocol Label List", "Data Type"=3, "Command"="BUS{SerialBus}:SYMB", "Access"=2, "Range Table"="", "Read Callback"="", "Write Callback"="", "Supported Models"="", "Instrument Options"="", "Flags"=0, "Help"="This function activates the label list to be used for decoding. The &apos;Label&apos; appear in the &apos;Decode results&apos; table and in the frame captions of the decoded signal.\n\nAvailable Repeated Capabilities:\nSerialBus: SB1, SB2, SB3, SB4\r\n\nRemote-control command(s):\nBUS<m>:SYMBols"}, {"Level"=2, "Class Only"=FALSE, "Identifier"="RSSCOPE_ATTR_PROTOCOL_LABEL_LIST_FILE", "Descriptive Name"="Protocol Label List File", "Data Type"=2, "Command"="BUS{SerialBus}:NEWL", "Access"=1, "Range Table"="", "Read Callback"="", "Write Callback"="", "Supported Models"="", "Instrument Options"="", "Flags"=0, "Help"="Loads a label list file.\n\nAvailable Repeated Capabilities:\nSerialBus: SB1, SB2, SB3, SB4\r\n\nRemote-control command(s):\nBUS<m>:NEWList"}, {"Level"=2, "Class Only"=FALSE, "Identifier"="RSSCOPE_ATTR_PROTOCOL_REFERENCE_LEVELS", "Descriptive Name"="Protocol Reference Levels", "Data Type"=4, "Command"="BUS{SerialBus}:SETR", "Access"=1, "Range Table"="", "Read Callback"="", "Write Callback"="", "Supported Models"="", "Instrument Options"="", "Flags"=0, "Help"="Executes the measurement of reference levels and sets the thresholds to the middle reference level of the measured amplitude.\n\nAvailable Repeated Capabilities:\nSerialBus: SB1, SB2, SB3, SB4\r\n\nRemote-control command(s):\nBUS<m>:SETReflevels"}, {"Level"=2, "Class Only"=FALSE, "Identifier"="RSSCOPE_ATTR_PROTOCOL_AUTOSET_THRESHOLD_AND_BITRATE", "Descriptive Name"="Protocol Autoset Threshold And Bitrate", "Data Type"=4, "Command"="BUS{SerialBus}:FAUT", "Access"=1, "Range Table"="", "Read Callback"="", "Write Callback"="", "Supported Models"="", "Instrument Options"="", "Flags"=0, "Help"="Starts software algorithms for determining the signal threshold levels and bitrate.\n\nAvailable Repeated Capabilities:\nSerialBus: SB1, SB2, SB3, SB4\r\n\nRemote-control command(s):\nBUS<m>:FAUToset"}, {"Level"=2, "Class Only"=TRUE, "Identifier"="", "Descriptive Name"="Export Protocol Results", "Data Type"=0, "Command"="", "Access"=0, "Range Table"="", "Read Callback"="", "Write Callback"="", "Supported Models"="", "Instrument Options"="", "Flags"=0, "Help"="You can export the results and all details of the selected protocol."}, {"Level"=3, "Class Only"=FALSE, "Identifier"="RSSCOPE_ATTR_PROTOCOL_EXPORT_INCLUDE_FRAME_TIMING", "Descriptive Name"="Protocol Export Include Frame Timing", "Data Type"=3, "Command"="BUS{SerialBus}:EXPR:TIME", "Access"=2, "Range Table"="", "Read Callback"="", "Write Callback"="", "Supported Models"="", "Instrument Options"="", "Flags"=0, "Help"="Includes the frame timing for the exported protocol results.\n\nAvailable Repeated Capabilities:\nSerialBus: SB1, SB2, SB3, SB4\r\n\nRemote-control command(s):\nBUS<m>:EXPResult:TIME"}, {"Level"=3, "Class Only"=FALSE, "Identifier"="RSSCOPE_ATTR_PROTOCOL_EXPORT_INCLUDE_DETAILS", "Descriptive Name"="Protocol Export Include Details", "Data Type"=3, "Command"="BUS{SerialBus}:EXPR:DET", "Access"=2, "Range Table"="", "Read Callback"="", "Write Callback"="", "Supported Models"="", "Instrument Options"="", "Flags"=0, "Help"="Includes the detailed results for all frames for the exported protocol results.\n\nAvailable Repeated Capabilities:\nSerialBus: SB1, SB2, SB3, SB4\r\n\nRemote-control command(s):\nBUS<m>:EXPResult:DETail"}, {"Level"=3, "Class Only"=FALSE, "Identifier"="RSSCOPE_ATTR_PROTOCOL_EXPORT_SAVE", "Descriptive Name"="Protocol Export Save", "Data Type"=2, "Command"="BUS{SerialBus}:EXPR:SAVE", "Access"=1, "Range Table"="", "Read Callback"="", "Write Callback"="", "Supported Models"="", "Instrument Options"="", "Flags"=0, "Help"="Saves the selected results to the indicated file.\n\nAvailable Repeated Capabilities:\nSerialBus: SB1, SB2, SB3, SB4\r\n\nRemote-control command(s):\nBUS<m>:EXPResult:SAVE"}, {"Level"=2, "Class Only"=TRUE, "Identifier"="", "Descriptive Name"="I2C", "Data Type"=0, "Command"="", "Access"=0, "Range Table"="", "Read Callback"="", "Write Callback"="", "Supported Models"="", "Instrument Options"="", "Flags"=0, "Help"="I2C (Inter-Integrated circuit bus) - decoding requires option R&S RTO-K1"}, {"Level"=3, "Class Only"=FALSE, "Identifier"="RSSCOPE_ATTR_PROTOCOL_I2C_TECHNOLOGY", "Descriptive Name"="Protocol I2C Technology", "Data Type"=0, "Command"="BUS{SerialBus}:I2C:TECH", "Access"=2, "Range Table"="rsscope_rngProtocolTechnology", "Read Callback"="", "Write Callback"="", "Supported Models"="", "Instrument Options"="", "Flags"=0, "Help"="Sets the threshold voltage clock and data lines as defined for various signal technologies.\n\nFor user defined values set to manual and use RSSCOPE_ATTR_PROTOCOL_I2C_THRESHOLD.\n\nAvailable Repeated Capabilities:\nSerialBus: SB1, SB2, SB3, SB4\r\n\nRemote-control command(s):\nBUS<m>:I2C:TECHnology"}, {"Level"=3, "Class Only"=FALSE, "Identifier"="RSSCOPE_ATTR_PROTOCOL_I2C_RW_BIT", "Descriptive Name"="Protocol I2C RW Bit", "Data Type"=0, "Command"="BUS{SerialBus}:I2C:RWB",
